vi "Gantry Vision Sandbox.vi"() -> ()   [LabVIEW 2011]
uses:
  Gantry Class.lvclass
panel:
  out "error out":errorcluster
  out "Image 2":T1(plugin-control)
  in  "stop":bool
  out "Image":T1(plugin-control)
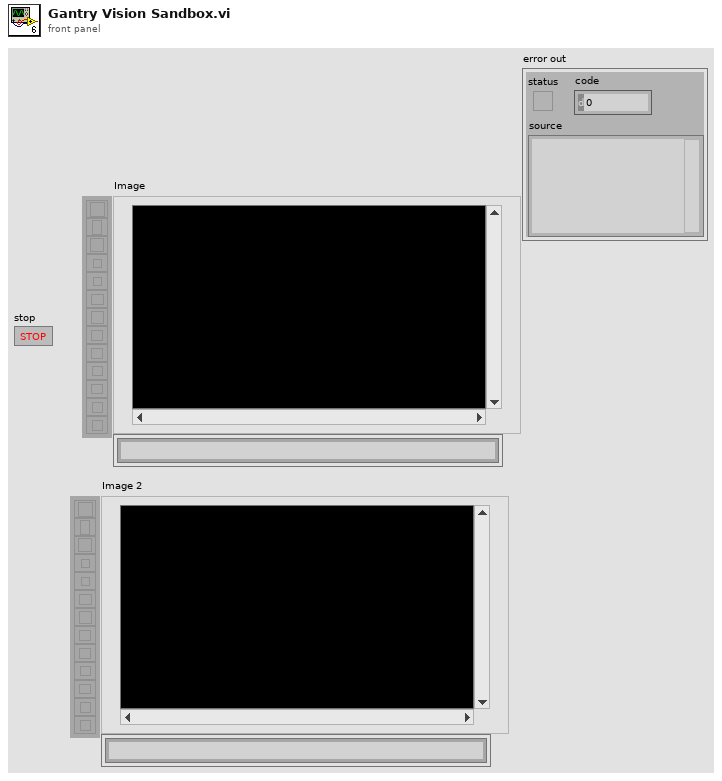
[diagram p1: front panel]
types:
  T1 = typedef "IMAQ Image.ctl" = refnum<image>
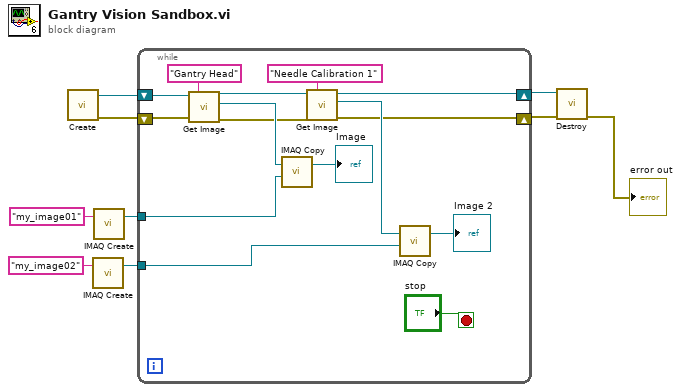
[diagram p0: block diagram]
diagram:
  n1 = call "Create.vi"() -> ("error out"=w8:errorcluster, "Gantry Class out"=w9:refnum<class "Gantry Class.lvclass">)  [unwired: 10 in]
  n2 = call "IMAQ Create"("Image Name"="my_image02") -> ("New Image"=w4:T1)  [unwired: 4 in, 1 out]
  n3 = call "IMAQ Create"("Image Name"="my_image01") -> ("New Image"=w6:T1)  [unwired: 4 in, 1 out]
  n4 = while {
    shift-right: [w17] -> w3
    shift-left: w9 -> [w24]
    shift-right: [w12] -> w2
    shift-left: w8 -> [w23]
    tunnel: w6 -> [w20]
    tunnel: w4 -> [w15]
    stop <- "stop" stop-if-true
    n5 = call "Get Image.vi"("error in (no error)"=w23, "Camera Name"="Gantry Head", "Gantry Class in"=w24) -> ("error out"=w13:errorcluster, "Image Out"=w21:T1, "Gantry Class out"=w18:refnum<class "Gantry Class.lvclass">)  [unwired: 6 in]
    n6 = call "IMAQ Copy"("Image Dst"=w20, "Image Src"=w21) -> ("Image Dst Out"=→"Image":T1)  [unwired: 4 in, 1 out]
    n7 = call "Get Image.vi"("error in (no error)"=w13, "Camera Name"="Needle Calibration 1", "Gantry Class in"=w18) -> ("error out"=w12:errorcluster, "Image Out"=w14:T1, "Gantry Class out"=w17:refnum<class "Gantry Class.lvclass">)  [unwired: 6 in]
    n8 = call "IMAQ Copy"("Image Dst"=w15, "Image Src"=w14) -> ("Image Dst Out"=→"Image 2":T1)  [unwired: 4 in, 1 out]
  }
  n9 = call "Destroy.vi"("error in (no error)"=w2, "Gantry Class in"=w3) -> ("error out"=→"error out":errorcluster)  [unwired: 9 in]
